vi "Logging Globale Variable.vi"() -> ()   [LabVIEW 2016]
panel:
  out "Integrator\nValue":dbl
  out "Actual Velocity":dbl
  out "Target Speed":dbl
  out "Velocity Error":dbl
  out "Break Voltage":dbl
  out "Throttle Voltage":dbl
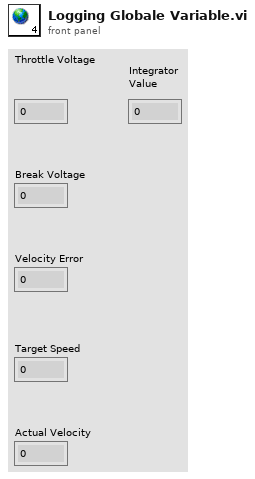
[diagram p1: front panel]
diagram:
